vi "overlay.vi"(0 "Image in":T2, 1 "classes":string[](array[string]), 2 "bboxes":T3(array[cluster]), 3 "scores":dbl[](array[numeric])) -> (7 "Image":T2)   [LabVIEW 2024]
uses:
  <vilib>/vision/Image Controls.llb/IMAQ Image.ctl
panel:
  out "Y Resolution":i32
  out "X Resolution":i32
  out "output cluster":T1
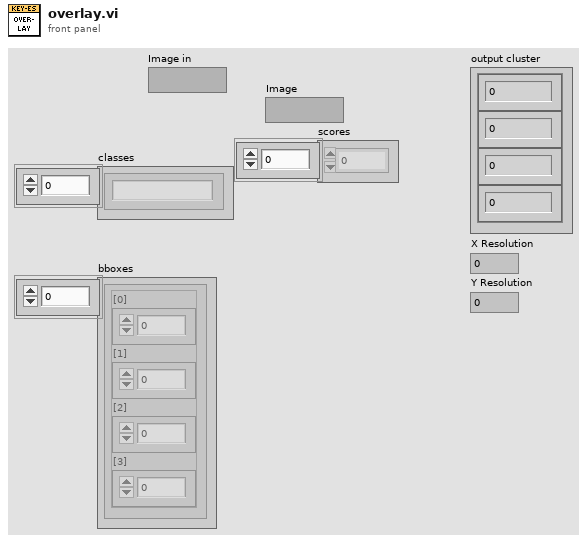
[diagram p1: front panel]
types:
  T1 = cluster{"Numeric":dbl, "Numeric":dbl, "Numeric":dbl, "Numeric":dbl}
  T2 = typedef "IMAQ Image.ctl" = refnum<image>
  T3 = cluster{"[0]":dbl, "[1]":dbl, "[2]":dbl, "[3]":dbl}[]
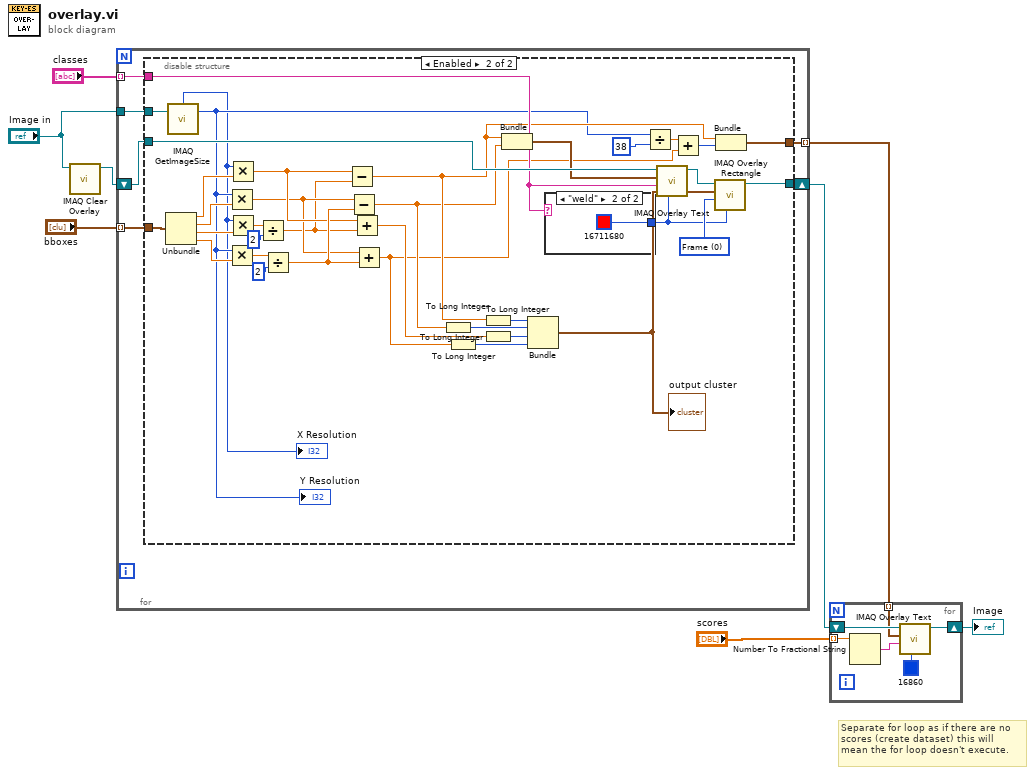
[diagram p0: block diagram]
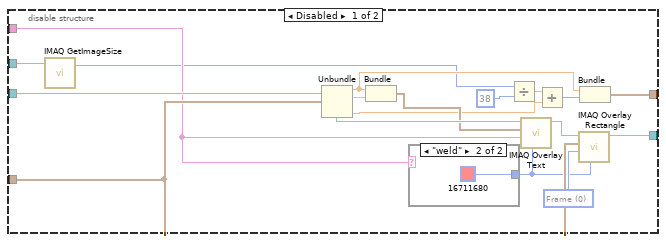
[diagram p2: hidden frame]
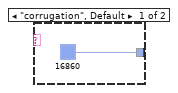
[diagram p3: hidden frame]
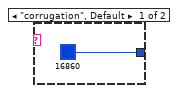
[diagram p4: hidden frame]
diagram:
  # "Separate for loop as if there are no\nscores (create dataset) this will\nmean the for loop doesn't execute."
  n1 = call "IMAQ Clear Overlay"("Image"="Image in") -> ("Image Out"=w2:T2)  [unwired: 9 in, 1 out]
  n2 = for {
    tunnel: "bboxes" -> [w13] mode=indexing
    shift-right: [w12] -> w5
    shift-left: w2 -> [w14]
    tunnel: "classes" -> [w10] mode=indexing
    tunnel: [w11] -> w3 mode=indexing
    tunnel: "Image in" -> [w9]
    n3 = disable-structure shown="Enabled" {
      disable-tunnel: w14 -> [w30 w68]
      disable-tunnel: w13 -> [w27 w66]
      disable-tunnel: [w24 w65] -> w12
      disable-tunnel: [w21 w36] -> w11
      disable-tunnel: w10 -> [w18 w61]
      disable-tunnel: w9 -> [w16 w59]
      frame Disabled {
        w31 = u32 0 items=["Frame", "Fill"] ("Drawing Mode (Frame)")
        n4 = call "IMAQ GetImageSize"("Image"=w16) -> ("Y Resolution"=w15:i32)  [unwired: 3 in, 2 out]
        n5 = Unbundle(w27) -> ("[0]"=w22:dbl, "[1]"=w28:dbl, "[3]"=w25:dbl)  [unwired: 1 out]
        n6 = Bundle("[0]"=w22, "[1]"=w28) -> (w26:cluster{"[0]":dbl, "[1]":dbl})  [unwired: 1 in]
        n7 = case shown="\"weld\"" w18 {
          tunnel: [u32 16860 ("Color") u32 16711680 ("Color")] -> w17
          frame "corrugation", Default {
          }
          frame "weld" {
          }
        }
        n8 = Divide(x=w15, y=38) -> (x/y=w20:dbl)
        n9 = call "IMAQ Overlay Text"("Text Color (black)"=w17, "String"=w18, "Origin"=w26, "Image"=w30) -> ("Image Out"=w29:T2)  [unwired: 6 in, 1 out]
        n10 = Add(x=w20, y=w25) -> (x+y=w23:i32)
        n11 = call "IMAQ Overlay Rectangle"("Color"=w17, "Drawing Mode (Frame)"=w31, "Rectangle"=w27, "Image"=w29) -> ("Image Out"=w24:T2)  [unwired: 6 in, 1 out]
        n12 = Bundle("[0]"=w22, w23) -> (w21:cluster{"[0]":dbl, i32})  [unwired: 1 in]
      }
      frame Enabled {
        w69 = u32 0 items=["Frame", "Fill"] ("Drawing Mode (Frame)")
        n13 = Unbundle(w66) -> ("[0]"=w58:dbl, "[1]"=w57:dbl, "[2]"=w56:dbl, "[3]"=w55:dbl)
        n14 = call "IMAQ GetImageSize"("Image"=w59) -> ("Y Resolution"=w35:i32, "X Resolution"=w34:i32)  [unwired: 3 in, 1 out]
        "X Resolution" <- w34
        "Y Resolution" <- w35
        n15 = Multiply(x=w35, y=w57) -> (x*y=w48:dbl)
        n16 = Multiply(x=w35, y=w55) -> (x*y=w51:dbl)
        n17 = Multiply(x=w34, y=w58) -> (x*y=w49:dbl)
        n18 = Multiply(x=w34, y=w56) -> (x*y=w54:dbl)
        n19 = Divide(x=w54, y=2) -> (x/y=w47:dbl)
        n20 = Divide(x=w51, y=2) -> (x/y=w50:dbl)
        n21 = Subtract(x=w49, y=w47) -> (x-y=w44:dbl)
        n22 = Subtract(x=w48, y=w50) -> (x-y=w42:dbl)
        n23 = Add(x=w49, y=w47) -> (x+y=w40:dbl)
        n24 = Add(x=w48, y=w50) -> (x+y=w37:dbl)
        n25 = To Long Integer(number=w42) -> (32bit integer=w41:i32)
        n26 = To Long Integer(number=w37) -> (32bit integer=w38:i32)
        n27 = To Long Integer(number=w44) -> (32bit integer=w43:i32)
        n28 = To Long Integer(number=w40) -> (32bit integer=w39:i32)
        n29 = Bundle(w44, w42) -> (w46:cluster{dbl, dbl})  [unwired: 1 in]
        n30 = Bundle(w43, w41, w39, w38) -> (w45:cluster{i32, i32, i32, i32})  [unwired: 1 in]
        "output cluster" <- w45
        n31 = case shown="\"weld\"" w61 {
          tunnel: [u32 16860 ("Color") u32 16711680 ("Color")] -> w60
          frame "corrugation", Default {
          }
          frame "weld" {
          }
        }
        n32 = Divide(x=w35, y=38) -> (x/y=w63:dbl)
        n33 = call "IMAQ Overlay Text"("Text Color (black)"=w60, "String"=w61, "Origin"=w46, "Image"=w68) -> ("Image Out"=w67:T2)  [unwired: 6 in, 1 out]
        n34 = Add(x=w63, y=w37) -> (x+y=w64:i32)
        n35 = call "IMAQ Overlay Rectangle"("Color"=w60, "Drawing Mode (Frame)"=w69, "Rectangle"=w45, "Image"=w67) -> ("Image Out"=w65:T2)  [unwired: 6 in, 1 out]
        n36 = Bundle(w44, w64) -> (w36:cluster{dbl, i32})  [unwired: 1 in]
      }
    }
  }
  n37 = for {
    tunnel: "scores" -> [w76] mode=indexing
    shift-right: [w74] -> w4
    shift-left: w5 -> [w75]
    tunnel: w3 -> [w73] mode=indexing
    n38 = Number To Fractional String(number=w76) -> (F-format string=w77:string)  [unwired: 3 in]
    n39 = call "IMAQ Overlay Text"("Text Color (black)"=u32 16860, "String"=w77, "Origin"=w73, "Image"=w75) -> ("Image Out"=w74:T2)  [unwired: 6 in, 1 out]
  }
  "Image" <- w4
